vi "find tag mapped to channel.vi"(7 "owner":string, 8 "error in":errorcluster, 10 "channel":refnum<class "TBM channel.lvclass">, 11 "engine configuration in":refnum<class "engine configuration.lvclass">) -> (0 "error out":errorcluster, 2 "tag":refnum<class "tag descriptor.lvclass">, 3 "engine configuration out":refnum<class "engine configuration.lvclass">)   [LabVIEW 2014, in "engine configuration.lvclass"]
doc: "For a given channel and its owner, this function will return the tag that is mapped to it."
uses:
  engine configuration.lvclass
  <vilib>/NI/Tag Bus Module Framework/channel/TBM channel.lvclass
  <vilib>/NI/Tag Bus/tag/tag descriptor.lvclass
  <vilib>/NI/Tag Bus/tag/tag descriptor.lvclass/tag descriptor.ctl
  engine configuration.lvclass/engine configuration.ctl
  <vilib>/NI/Tag Bus/tag/read tag name.vi
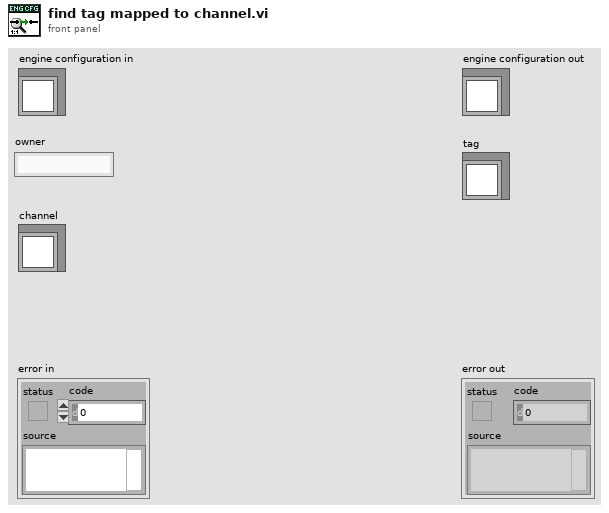
[diagram p1: front panel]
types:
  T1 = typedef "tag bus.lvlib/tag descriptor.lvclass/Data Type.ctl" = enum16{"Double", "Single", "I64", "I32", "I16", "I8", "U64", "U32", "U16", "U8", "Boolean", "String", "Array of Double", "Array of Single", "Array of I64", "Array of I32", "Array of I16", "Array of I8", "Array of U64", "Array of U32", "Array of U16", "Array of U8", "Array of Boolean", "Array of String"}
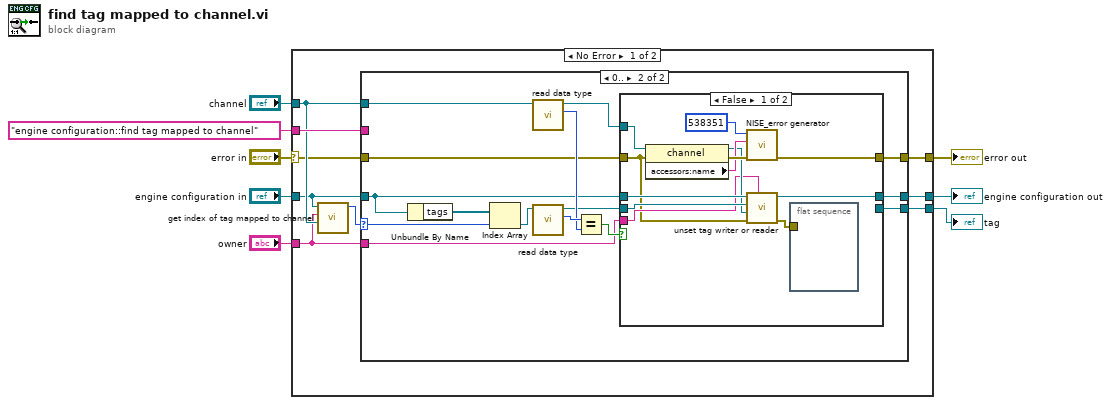
[diagram p0: block diagram]
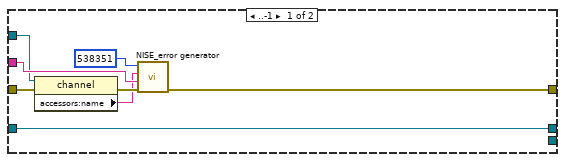
[diagram p2: hidden frame]
diagram:
  n1 = case shown="No Error" "error in" {
    selector: "error in" -> [w12 w57]
    tunnel: [w16 w57] -> w7
    tunnel: [w10 w56] -> w5
    tunnel: "engine configuration in" -> [w11 w56]
    tunnel: "owner" -> [w9 _]
    tunnel: "channel" -> [w13 _]
    tunnel: [w17 _] -> w2
    tunnel: "engine configuration::find tag mapped to channel" ("source") -> [w15 _]
    frame No Error {
      n2 = call-dynamic "get index of tag mapped to channel.vi"("channel"=w13, "owner"=w9, "engine configuration in"=w11) -> ("tag index"=w14:i32)  [unwired: 8 in]
      n3 = case shown="0.." w14 {
        selector: w14 -> [_ w39]
        tunnel: [_ w34] -> w17
        tunnel: w12 -> [w20 w32]
        tunnel: [w24 w31] -> w16
        tunnel: w15 -> [w23 _]
        tunnel: w13 -> [w19 w38]
        tunnel: w11 -> [w18 w26]
        tunnel: [w18 w29] -> w10
        tunnel: w9 -> [_ w28]
        frame ..-1 {
          n4 = property class="channel"(reference=w19, error in=w20) -> (error out=w22:errorcluster, "accessors:name"=w21:string)  [unwired: 1 out]
          n5 = call <vilib>:"NISE_error generator.vi"("error in"=w22, "source"=w23, "append error message"=w21, "error code (0)"=538351) -> ("error out"=w24:errorcluster)  [unwired: 5 in]
        }
        frame 0.. {
          n6 = Unbundle By Name(w26) -> ("tags"=w27:refnum<class "tag descriptor.lvclass">[])
          n7 = Index Array(array=w27, index=w39) -> (element=w40:refnum<class "tag descriptor.lvclass">)
          n8 = call <vilib>:"read data type.vi"("system tag in"=w38) -> ("data type"=w36:T1, "system tag out"=w30:refnum<class "TBM channel.lvclass">)  [unwired: 8 in, 1 out]
          n9 = call <vilib>:"read data type.vi"("system tag in"=w40) -> ("data type"=w37:T1, "system tag out"=w33:refnum<class "tag descriptor.lvclass">)  [unwired: 8 in, 1 out]
          n10 = Equal?(x=w37, y=w36) -> (x = y?=w35:bool)
          n11 = case shown="False" w35 {
            tunnel: [_ w55] -> w34
            tunnel: w33 -> [w44 w55]
            tunnel: w32 -> [w41 w54]
            tunnel: [w49 w54] -> w31
            tunnel: w30 -> [w48 _]
            tunnel: w26 -> [w46 w53]
            tunnel: [w45 w53] -> w29
            tunnel: w28 -> [w42 _]
            frame False {
              n12 = property class="channel"(reference=w48, error in=w41) -> (reference out=w43:refnum<class "TBM channel.lvclass">, error out=w51:errorcluster, "accessors:name"=w50:string)
              n13 = call <vilib>:"NISE_error generator.vi"("error in"=w51, "append error message"=w50, "error code (0)"=538351) -> ("error out"=w49:errorcluster)  [unwired: 6 in]
              n14 = call-dynamic "unset tag writer or reader.vi"("module GUID"=w42, "error in"=w41, "channel"=w43, "tag descriptor"=w44, "engine configuration in"=w46) -> ("error out"=w47:errorcluster, "engine configuration out"=w45:refnum<class "engine configuration.lvclass">)  [unwired: 5 in]
              n15 = flat-sequence {
                tunnel: w47 -> [_]
                frame #0 {
                }
              }
            }
            frame True {
            }
          }
        }
      }
    }
    frame Error {
    }
  }
  "error out" <- w7
  "engine configuration out" <- w5
  "tag" <- w2
